vi "MSEncoder Case-45-FGen.vi"(8 "error in (no error)":errorcluster, 9 "ParamValIn":variant, 11 "MSEncoder in":refnum<class "MSEncoder.lvclass">) -> (0 "error out":errorcluster, 3 "MSEncoder out":refnum<class "MSEncoder.lvclass">)   [LabVIEW 2018, in "MSEncoder.lvclass"]
uses:
  MSEncoder.lvclass
  Ctl/MSEditorParam FGen.ctl
  MSEncoder.lvclass/MSEncoder.ctl
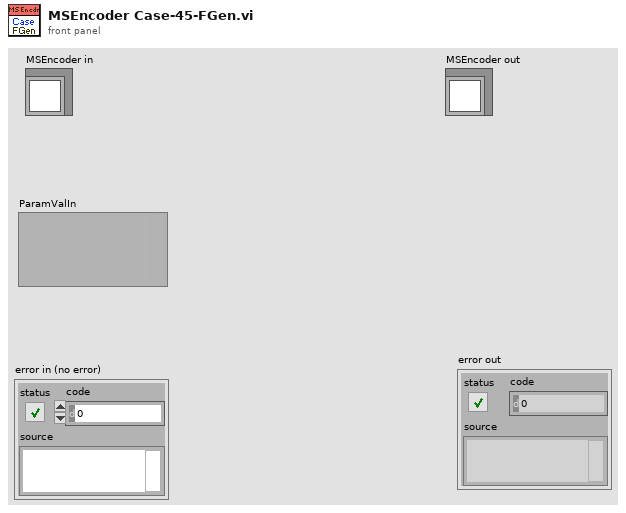
[diagram p1: front panel]
types:
  T1 = typedef "MSEditorParam FGen.ctl" = cluster{"amp":ext, "freq":ext}
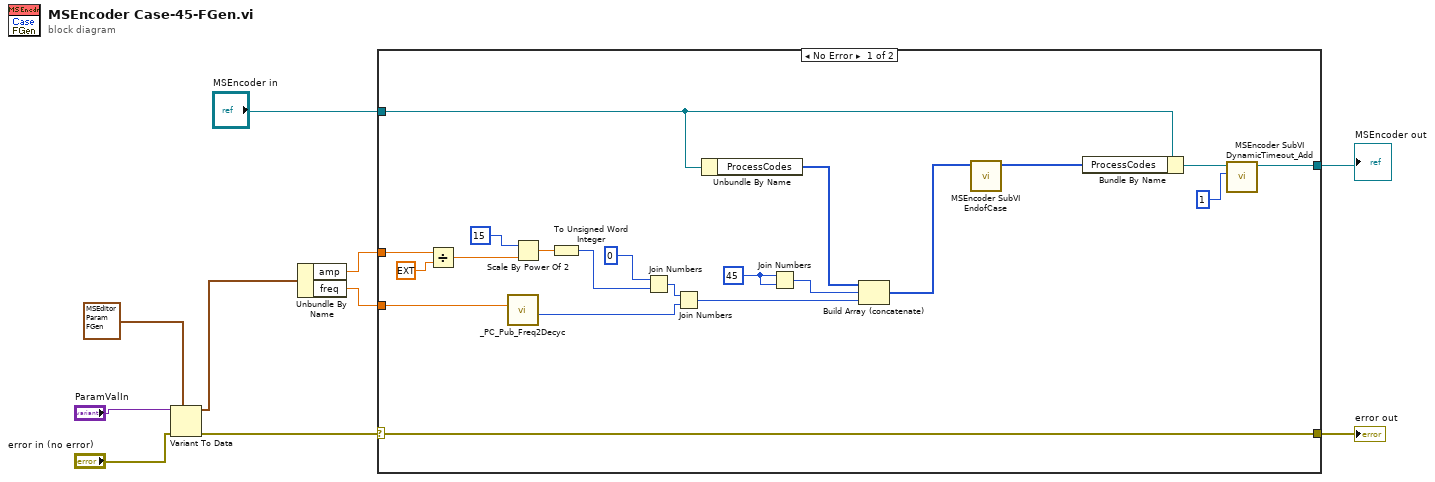
[diagram p0: block diagram]
diagram:
  n1 = Variant To Data(error in="error in (no error)", type=T1 {"amp"=0.001, "freq"=0.01} ("ParamValueType"), Variant="ParamValIn") -> (data=w3:T1, error out=w2:errorcluster)
  n2 = Unbundle By Name(w3) -> ("amp"=w9:ext, "freq"=w8:ext)
  n3 = case shown="No Error" w2 {
    selector: w2 -> [w30 w33]
    tunnel: "MSEncoder in" -> [w29 w32]
    tunnel: [w30 w33] -> w10
    tunnel: [w13 w32] -> w7
    tunnel: w9 -> [w11 _]
    tunnel: w8 -> [w15 _]
    frame No Error {
      w27 = u32 45
      n4 = Divide(x=w11, y=ext 3.0 ("x")) -> (x/y=w17:ext)
      n5 = call "_PC_Pub_Freq2Decyc.vi"("Freq"=w15) -> ("Decyc*2^32"=w20:u32)  [unwired: 4 in, 4 out]
      n6 = Scale By Power Of 2(n=i16 15, x=w17) -> (x*2^n=w23:ext)
      n7 = To Unsigned Word Integer(number=w23) -> (unsigned 16bit integer=w22:u16)
      n8 = Join Numbers(hi=u16 0, lo=w22) -> ((hi.lo)=w21:u32)
      n9 = Join Numbers(hi=w21, lo=w20) -> ((hi.lo)=w18:u64)
      n10 = Unbundle By Name(w29) -> ("ProcessCodes"=w31:u64[])
      n11 = Join Numbers(hi=w27, lo=w27) -> ((hi.lo)=w26:u64)
      n12 = Build Array (concatenate)(w31, w26, w18) -> (w25:u64[])
      n13 = call "MSEncoder SubVI EndofCase.vi"("Case codes"=w25) -> ("Case codes with end"=w28:u64[])  [unwired: 9 in, 1 out]
      n14 = Bundle By Name(cluster=w29, "ProcessCodes"=w28) -> (w14:refnum<class "MSEncoder.lvclass">)
      n15 = call "MSEncoder SubVI DynamicTimeout_Add.vi"("Timeout_ms"=1, "MSEncoder"=w14) -> ("MSEncoder"=w13:refnum<class "MSEncoder.lvclass">)  [unwired: 8 in, 1 out]
    }
    frame Error {
    }
  }
  "error out" <- w10
  "MSEncoder out" <- w7
